vi "ConfigureCheckStepNameLengthDialog.vi"(6 "error in (no error)":errorcluster, 8 "Maximum Step Name Length:":i32, 9 "RuleConfigurationContext in":refnum<k7>) -> (0 "error out":errorcluster, 1 "OKButtonClicked":bool, 2 "Maximum Step Name Length out":i32, 3 "RuleConfigurationContext out":refnum<k7>)   [LabVIEW 2011]
panel:
  in  "Cancel":bool
  in  "OK":bool
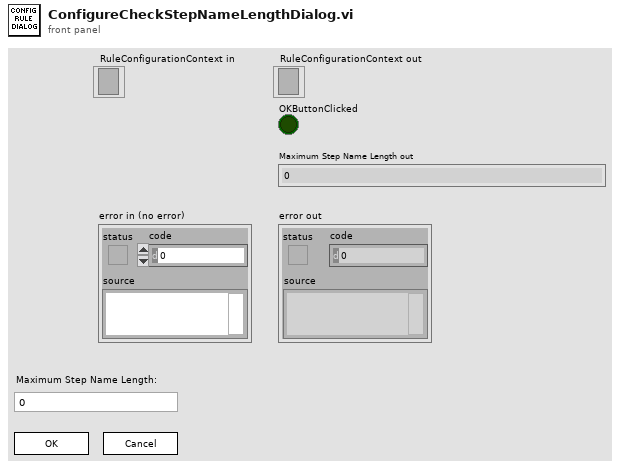
[diagram p1: front panel]
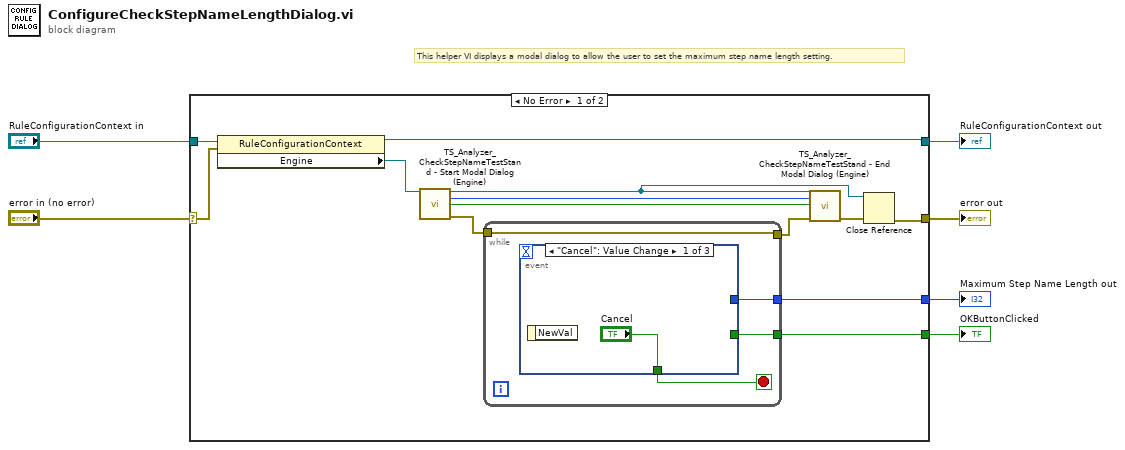
[diagram p0: block diagram]
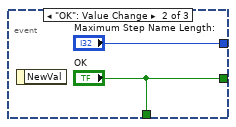
[diagram p2: hidden frame]
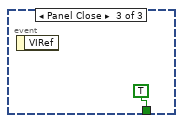
[diagram p3: hidden frame]
diagram:
  # "This helper VI displays a modal dialog to allow the user to set the maximum step name length setting."
  n1 = case shown="No Error" "error in (no error)" {
    selector: "error in (no error)" -> [w12 w29]
    tunnel: [w9 w29] -> w6
    tunnel: "RuleConfigurationContext in" -> [w17 w28]
    tunnel: [w16 _] -> w4
    tunnel: [w15 _] -> w3
    tunnel: [w11 w28] -> w1
    frame No Error {
      n2 = property class="RuleConfigurationContext"(reference=w17, error in=w12) -> (reference out=w11:refnum<k7>, "Engine"=w7:refnum<k7>)  [unwired: 1 out]
      n3 = call "TS_Analyzer_CheckStepNameTestStand - Start Modal Dialog (Engine).vi"("Engine in"=w7) -> ("Engine out"=w8:refnum<k7>, "Modal ID"=w19:i32, "VI Originally Open"=w18:bool, "error out"=w14:errorcluster)  [unwired: 10 in, 1 out]
      n4 = while {
        tunnel: [w22] -> w16
        tunnel: [w21] -> w15
        tunnel: w14 -> [w20]
        tunnel: [w20] -> w13
        stop <- w23 stop-if-true
        n5 = event shown="[0] \"Cancel\": Value Change" {
          selector: _ -> [_ _ _]
          dyn-events: _ -> [_ _ _]
          timeout: _ -> [_ _ _]
          tunnel: ["Cancel" "OK" TRUE ("OK")] -> w23
          tunnel: [_ "OK" _] -> w22
          tunnel: [_ "Maximum Step Name Length:" _] -> w21
          event "Cancel": Value Change {
            n6 = event-data() -> ()  [unwired: 2 out]
          }
          event "OK": Value Change {
            n7 = event-data() -> ()  [unwired: 2 out]
          }
          event Panel Close {
            n8 = event-data() -> ()  [unwired: 2 out]
          }
        }
      }
      n9 = call "TS_Analyzer_CheckStepNameTestStand - End Modal Dialog (Engine).vi"("Engine"=w8, "Modal ID"=w19, "VI Originally Open"=w18, "error in (no error)"=w13) -> ("error out"=w10:errorcluster)  [unwired: 11 in]
      n10 = Close Reference(reference=w8, error in (no error)=w10) -> (error out=w9:errorcluster)
    }
    frame Error {
    }
  }
  "error out" <- w6
  "OKButtonClicked" <- w4
  "Maximum Step Name Length out" <- w3
  "RuleConfigurationContext out" <- w1
